vi "Launch Guest Manager.vi"(0 "Rooms Manager Model in":refnum<class "Rooms Manager Model.lvclass">, 5 "Check-in":bool, 11 "error in (no error)":errorcluster) -> (4 "Rooms Manager Model out":refnum<class "Rooms Manager Model.lvclass">, 15 "error out":errorcluster)   [LabVIEW 2023, in "Rooms Manager Model.lvlib" / "Rooms Manager Model.lvclass"]
uses:
  Rooms Manager Model.lvclass
  Rooms Manager Model.lvclass/Rooms Manager Model.ctl
  <vilib>/ActorFramework/Actor/Actor.lvclass
  Guest Manager Model/Guest Manager Model/Guest Manager Model.lvclass
  Guest Manager Model/Guest Manager Model Messages/Select Operation Msg/Select Operation Msg.lvclass
  C:/Users/bhaghyaraj/Trainings/NI Actor Framework/SDLC/Model Base/Model Base/Model Base.lvclass
  C:/Program Files/National Instruments/LabVIEW 2023/vi.lib/ActorFramework/Actor/Actor.lvclass
  C:/Users/bhaghyaraj/Trainings/NI Actor Framework/SDLC/Interfaces/Model Base/Incoming Model Base Interface.lvclass
  C:/Users/bhaghyaraj/Trainings/NI Actor Framework/SDLC/Rooms Manager Model/Rooms Manager Model/Rooms Manager Model.lvclass
  C:/Users/bhaghyaraj/Trainings/NI Actor Framework/SDLC/Interfaces/Rooms Manager Model/Incoming Rooms Manager Model Interface.lvclass
  Rooms Manager Model Messages/Request Check-out Details Msg/Request Check-out Details Msg.lvclass
  C:/Users/bhaghyaraj/Trainings/NI Actor Framework/SDLC/Guest Manager Model/Guest Manager Model/Guest Manager Model.lvclass
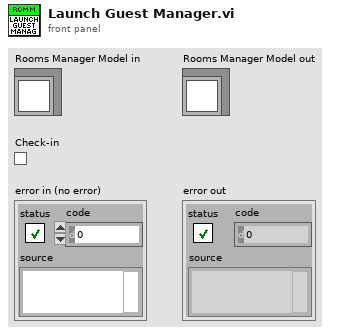
[diagram p1: front panel]
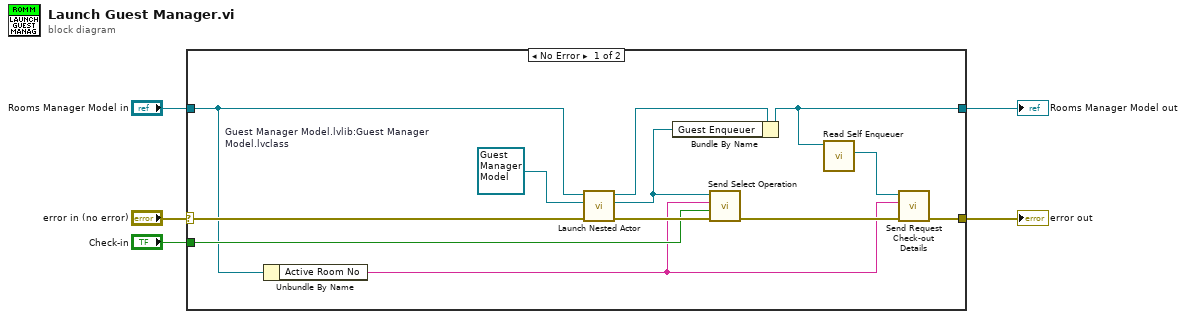
[diagram p0: block diagram]
diagram:
  n1 = case shown="No Error" "error in (no error)" {
    selector: "error in (no error)" -> [w17 w19]
    tunnel: [w11 w19] -> w4
    tunnel: [w9 w18] -> w2
    tunnel: "Rooms Manager Model in" -> [w7 w18]
    tunnel: "Check-in" -> [w8 _]
    frame No Error {
      w15 = refnum<class "Guest Manager Model.lvclass"> refnum  # Guest Manager Model.lvlib:Guest Manager Model.lvclass
      n2 = Unbundle By Name(w7) -> ("Active Room No"=w6:string)
      n3 = call <vilib>:"Launch Nested Actor.vi"("error in (no error)"=w17, "Nested Actor"=w15, "Caller Actor in"=w7) -> ("error out"=w14:errorcluster, "Nested Actor's Enqueuer"=w13:refnum<class "Message Enqueuer.lvclass">, "Caller Actor out"=w16:refnum<class "Rooms Manager Model.lvclass">)  [unwired: 6 in]
      n4 = Bundle By Name(cluster=w16, "Guest Enqueuer"=w13) -> (w9:refnum<class "Rooms Manager Model.lvclass">)
      n5 = call "Send Select Operation.vi"("error in (no error)"=w14, "Check-in"=w8, "Room No"=w6, "Message Enqueuer"=w13) -> ("error out"=w12:errorcluster)  [unwired: 6 in, 1 out]
      n6 = call <vilib>:"Read Self Enqueuer.vi"("Actor"=w9) -> ("Self Enqueuer"=w10:refnum<class "Message Enqueuer.lvclass">)  [unwired: 10 in]
      n7 = call "Send Request Check-out Details.vi"("error in (no error)"=w12, "Room No"=w6, "Message Enqueuer"=w10) -> ("error out"=w11:errorcluster)  [unwired: 7 in, 1 out]
    }
    frame Error {
    }
  }
  "error out" <- w4
  "Rooms Manager Model out" <- w2
